vi "Read Position.vi"(8 "error in (no error)":errorcluster, 11 "VISA resource name":refnum<visa-resource-name>) -> (0 "error out":errorcluster, 1 "Longitude (ddmm.mmmm)":dbl format="%_8g", 2 "Lattitude (ddmm.mmmm)":dbl format="%_8g", 3 "VISA resource name out":refnum<visa-resource-name>, 4 "Magnetic Variation (degrees)":dbl format="%_4g", 5 "UTC Time":timestamp, 6 "Speed over ground (knots)":dbl format="%_3g", 7 "GPS Data Valid?":bool)   [LabVIEW 2012, in "USGlobalSat.lvlib"]
uses:
  USGlobalSat.lvlib
panel:
  in  "date time rec":T1
  out "Local Time":timestamp
  in  "UTC Time Zone":i32=-5
  out "Lattitude North/South":string
  out "Longitude East/West":string
  out "Course over ground (degrees)":dbl format="%_4g"
  out "Variation East/West":string
  in  "Cluster":T2 {"Course over ground (degrees)" format="%_4g"; "Speed over ground (knots)" format="%_3g"; "Magnetic Variation (degrees)" format="%_4g"; "Longitude (ddmm.mmmm)" format="%_8g"; "Lattitude (ddmm.mmmm)" format="%_8g"}
  out "GPS Data":T2 {"Course over ground (degrees)" format="%#.6g"; "Speed over ground (knots)" format="%#.6g"; "Magnetic Variation (degrees)" format="%#.6g"; "Longitude (ddmm.mmmm)" format="%#.6g"; "Lattitude (ddmm.mmmm)" format="%#.6g"}
  out "String Read":string="\n"
  out "Bytes read":u32
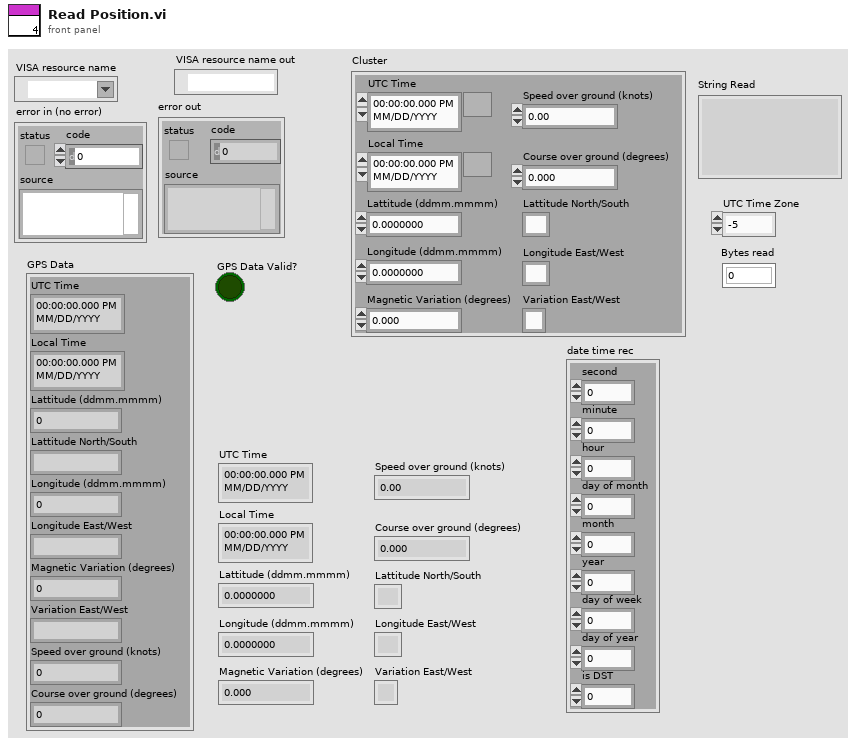
[diagram p1: front panel]
types:
  T1 = cluster{"second":i32, "minute":i32, "hour":i32, "day of month":i32, "month":i32, "year":i32, "day of week":i32, "day of year":i32, "is DST":i32}
  T2 = cluster{"UTC Time":timestamp, "Local Time":timestamp, "Lattitude (ddmm.mmmm)":dbl, "Lattitude North/South":string, "Longitude (ddmm.mmmm)":dbl, "Longitude East/West":string, "Magnetic Variation (degrees)":dbl, "Variation East/West":string, "Speed over ground (knots)":dbl, "Course over ground (degrees)":dbl}
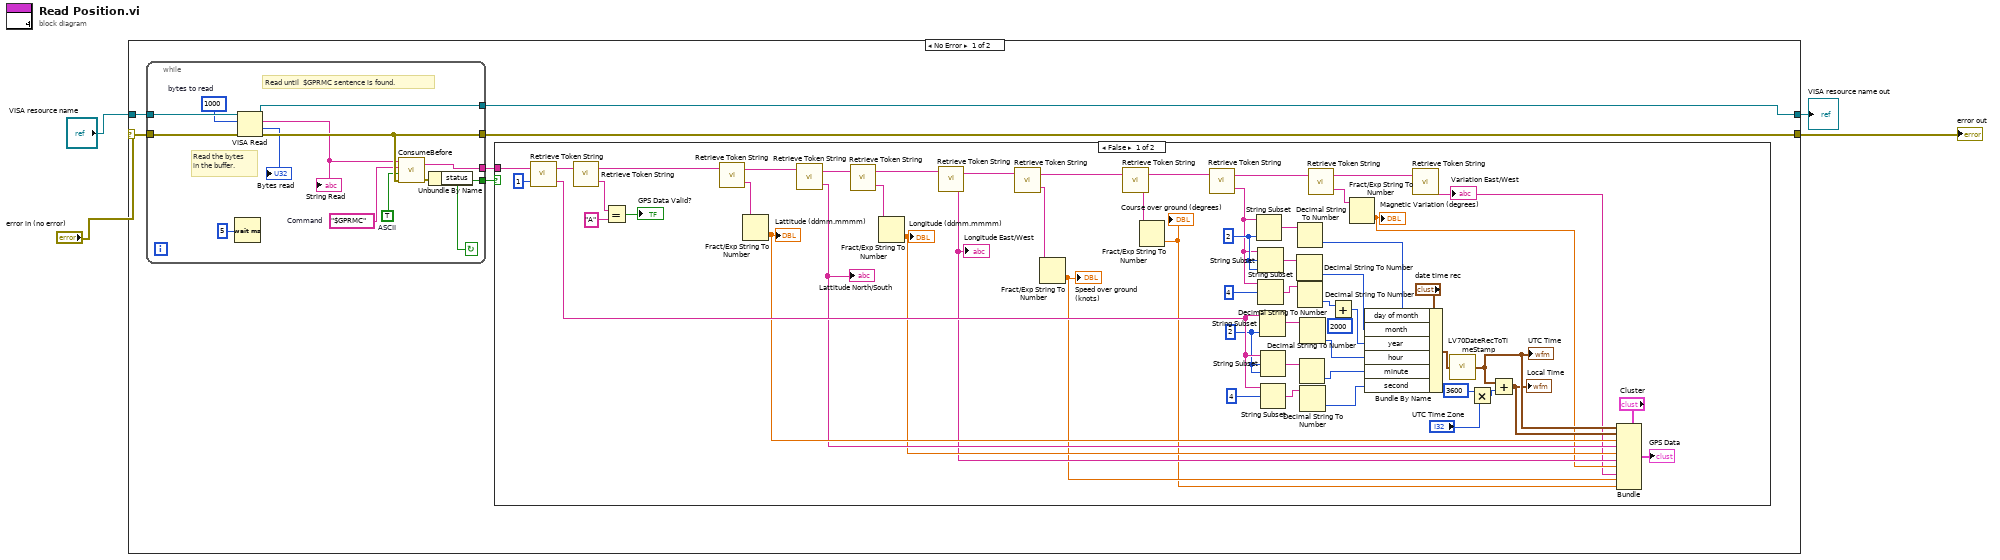
[diagram p0: block diagram]
diagram:
  n1 = case shown="No Error" "error in (no error)" {
    selector: "error in (no error)" -> [w7 w81]
    tunnel: "VISA resource name" -> [w10 w82]
    tunnel: [w9 w82] -> w1
    tunnel: [w8 w81] -> w2
    frame No Error {
      n2 = while {
        tunnel: w10 -> [w23]
        tunnel: [w22] -> w9
        tunnel: [w21] -> w8
        tunnel: w7 -> [w20]
        tunnel: [w16] -> w6
        tunnel: [w12] -> w5
        stop <- w12 continue-if-true
        w14 = u32 1000  # bytes to read
        w19 = "$GPRMC"  # Command
        w18 = TRUE  # ASCII
        # "Read until  $GPRMC sentence is found."
        # "Read the bytes\nin the buffer."
        n3 = Wait (ms)(milliseconds to wait=u32 5 ("millisecond multiple")) -> ()  [unwired: 1 out]
        n4 = VISA Read(VISA resource name=w23, byte count=w14, error in (no error)=w20) -> (VISA resource name out=w22:refnum<visa-resource-name>, read buffer=w17:string, return count=→"Bytes read":u32, error out=w21:errorcluster)
        "String Read" <- w17
        n5 = call <vilib>:"ConsumeBefore.vi"("error in"=w21, "ASCII"=w18, "Before"=w19, "Response String In"=w17) -> ("error out"=w15:errorcluster, "Response String Out"=w16:string)
        n6 = Unbundle By Name(w15) -> ("status"=w12:bool)
      }
      n7 = case shown="False" w5 {
        tunnel: w6 -> [w78 _]
        frame False {
          w46 = 2 ("length (rest)")
          w68 = 2 ("length (rest)")
          n8 = call "Retrieve Token String.vi"("Offset (0)"=1, "input string"=w78) -> ("token string"=w75:string, "output string"=w76:string)
          n9 = call "Retrieve Token String.vi"("input string"=w76) -> ("token string"=w80:string, "output string"=w74:string)  [unwired: 1 in]
          n10 = Equal?(x=w80, y="A") -> (x = y?=→"GPS Data Valid?":bool)
          n11 = call "Retrieve Token String.vi"("input string"=w74) -> ("token string"=w59:string, "output string"=w58:string)  [unwired: 1 in]
          n12 = Fract/Exp String To Number(string=w59) -> (number=w33:dbl)  [unwired: 3 in, 1 out]
          "Lattitude (ddmm.mmmm)" <- w33
          n13 = call "Retrieve Token String.vi"("input string"=w58) -> ("token string"=w32:string, "output string"=w57:string)  [unwired: 1 in]
          "Lattitude North/South" <- w32
          n14 = call "Retrieve Token String.vi"("input string"=w57) -> ("token string"=w56:string, "output string"=w55:string)  [unwired: 1 in]
          n15 = Fract/Exp String To Number(string=w56) -> (number=w31:dbl)  [unwired: 3 in, 1 out]
          "Longitude (ddmm.mmmm)" <- w31
          n16 = call "Retrieve Token String.vi"("input string"=w55) -> ("token string"=w30:string, "output string"=w54:string)  [unwired: 1 in]
          "Longitude East/West" <- w30
          n17 = call "Retrieve Token String.vi"("input string"=w54) -> ("token string"=w53:string, "output string"=w52:string)  [unwired: 1 in]
          n18 = Fract/Exp String To Number(string=w53) -> (number=w27:dbl)  [unwired: 3 in, 1 out]
          "Speed over ground (knots)" <- w27
          n19 = call "Retrieve Token String.vi"("input string"=w52) -> ("token string"=w51:string, "output string"=w50:string)  [unwired: 1 in]
          n20 = Fract/Exp String To Number(string=w51) -> (number=w26:dbl)  [unwired: 3 in, 1 out]
          "Course over ground (degrees)" <- w26
          n21 = call "Retrieve Token String.vi"("input string"=w50) -> ("token string"=w44:string, "output string"=w38:string)  [unwired: 1 in]
          n22 = String Subset(string=w44, length (rest)=w46) -> (substring=w45:string)  [unwired: 1 in]
          n23 = String Subset(string=w44, offset (0)=w46, length (rest)=w46) -> (substring=w47:string)
          n24 = String Subset(string=w44, offset (0)=4) -> (substring=w49:string)  [unwired: 1 in]
          n25 = String Subset(string=w75, length (rest)=w68) -> (substring=w72:string)  [unwired: 1 in]
          n26 = String Subset(string=w75, offset (0)=w68, length (rest)=w68) -> (substring=w66:string)
          n27 = String Subset(string=w75, offset (0)=4) -> (substring=w64:string)  [unwired: 1 in]
          n28 = Decimal String To Number(string=w47) -> (number=w42:i32)  [unwired: 2 in, 1 out]
          n29 = Decimal String To Number(string=w45) -> (number=w43:i32)  [unwired: 2 in, 1 out]
          n30 = Decimal String To Number(string=w49) -> (number=w41:i32)  [unwired: 2 in, 1 out]
          n31 = Decimal String To Number(string=w66) -> (number=w67:i32)  [unwired: 2 in, 1 out]
          n32 = Decimal String To Number(string=w72) -> (number=w69:i32)  [unwired: 2 in, 1 out]
          n33 = Decimal String To Number(string=w64) -> (number=w63:i32)  [unwired: 2 in, 1 out]
          n34 = call "Retrieve Token String.vi"("input string"=w38) -> ("token string"=w37:string, "output string"=w36:string)  [unwired: 1 in]
          n35 = Add(x=w41, y=2000) -> (x+y=w39:i32)
          n36 = Fract/Exp String To Number(string=w37) -> (number=w29:dbl)  [unwired: 3 in, 1 out]
          "Magnetic Variation (degrees)" <- w29
          n37 = Bundle By Name(cluster="date time rec", "day of month"=w43, "month"=w42, "year"=w39, "hour"=w69, "minute"=w67, "second"=w63) -> (w71:T1)
          n38 = call "Retrieve Token String.vi"("input string"=w36) -> ("token string"=w28:string)  [unwired: 1 in, 1 out]
          "Variation East/West" <- w28
          n39 = call <vilib>:"LV70DateRecToTimeStamp.vi"("date time rec"=w71) -> ("Time Stamp"=w35:timestamp)
          "UTC Time" <- w35
          n40 = Multiply(x=3600 ("number"), y="UTC Time Zone") -> (x*y=w60:i32)
          n41 = Add(x=w35, y=w60) -> (x+y=w34:timestamp)
          "Local Time" <- w34
          n42 = Bundle(cluster="Cluster", "UTC Time"=w35, "Local Time"=w34, "Lattitude (ddmm.mmmm)"=w33, "Lattitude North/South"=w32, "Longitude (ddmm.mmmm)"=w31, "Longitude East/West"=w30, "Magnetic Variation (degrees)"=w29, "Variation East/West"=w28, "Speed over ground (knots)"=w27, "Course over ground (degrees)"=w26) -> (→"GPS Data":T2)
        }
        frame True {
        }
      }
    }
    frame Error {
    }
  }
  "error out" <- w2
  "VISA resource name out" <- w1
